vi "IMAQdx Serial Read.vi"(7 "Timeout (ms)":u32=1000, 8 "error in":errorcluster, 11 "Session In":T1) -> (0 "error out":errorcluster, 2 "Data":string, 3 "Session Out":T1)   [LabVIEW 2020, in "NI_Vision_Acquisition_Software.lvlib"]
doc: "Reads in data from the serial port on image acquisition devices that support serial communication."
uses:
  NI_Vision_Acquisition_Software.lvlib
  IMAQdx.ctl
  niimaqdx.dll
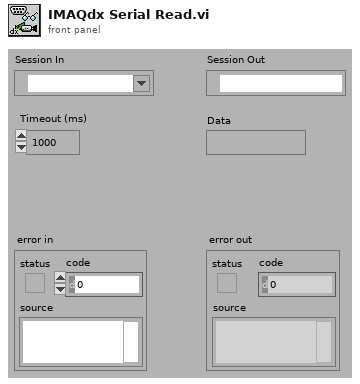
[diagram p1: front panel]
types:
  T1 = typedef "IMAQdx.ctl" = refnum<k21>
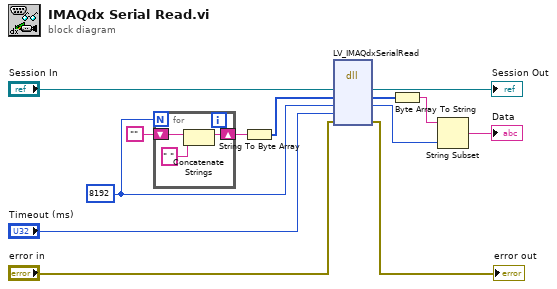
[diagram p0: block diagram]
diagram:
  w11 = u32 8192
  n1 = for {
    N: w11 -> [_]
    shift-right: [w15] -> w10
    shift-left: "" -> [w16]
    n2 = Concatenate Strings(w16, " ") -> (w15:string)
  }
  n3 = String To Byte Array(string=w10) -> (unsigned byte array=w9:u8[])
  n4 = dll-call lib="niimaqdx.dll" fn="LV_IMAQdxSerialRead"("refnum"="Session In", "StringToRead"=w9, "StringSize"=w11, "Timeout"="Timeout (ms)", "error"="error in") -> ("refnum"=→"Session Out":T1, "StringToRead"=w8:u8[], "StringSize"=w6:u32, "error"=→"error out":errorcluster)  [unwired: 4 in, 3 out]
  n5 = Byte Array To String(unsigned byte array=w8) -> (string=w1:string)
  n6 = String Subset(string=w1, length (rest)=w6) -> (substring=→"Data":string)  [unwired: 1 out]
